vi "convert type defs to channels.vi"() -> (0 "error out":errorcluster, 3 "Array out":refnum<class "TBM channel.lvclass">[](array[class]))   [LabVIEW 2013, in "fixed channel tag bus module configuration.lvclass"]
uses:
  fixed channel tag bus module configuration.lvclass
  <vilib>/NI/Tag Bus Module Framework/channel/TBM channel.lvclass
  <vilib>/NI/Tag Bus Module Framework/channel/channel classification.ctl
  <vilib>/regexp/Match Regular Expression.xnode
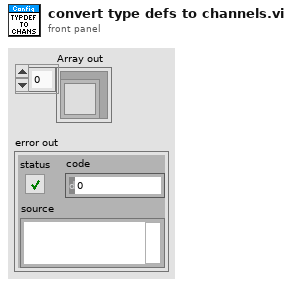
[diagram p1: front panel]
types:
  T1 = typedef "TBM channel.lvclass/channel classification.ctl" = enum16{"input data", "output data", "processing parameter", "processing result"}
  T2 = typedef "tag bus.lvlib/tag descriptor.lvclass/Data Type.ctl" = enum16{"Double", "Single", "I64", "I32", "I16", "I8", "U64", "U32", "U16", "U8", "Boolean", "String", "Array of Double", "Array of Single", "Array of I64", "Array of I32", "Array of I16", "Array of I8", "Array of U64", "Array of U32", "Array of U16", "Array of U8", "Array of Boolean", "Array of String"}
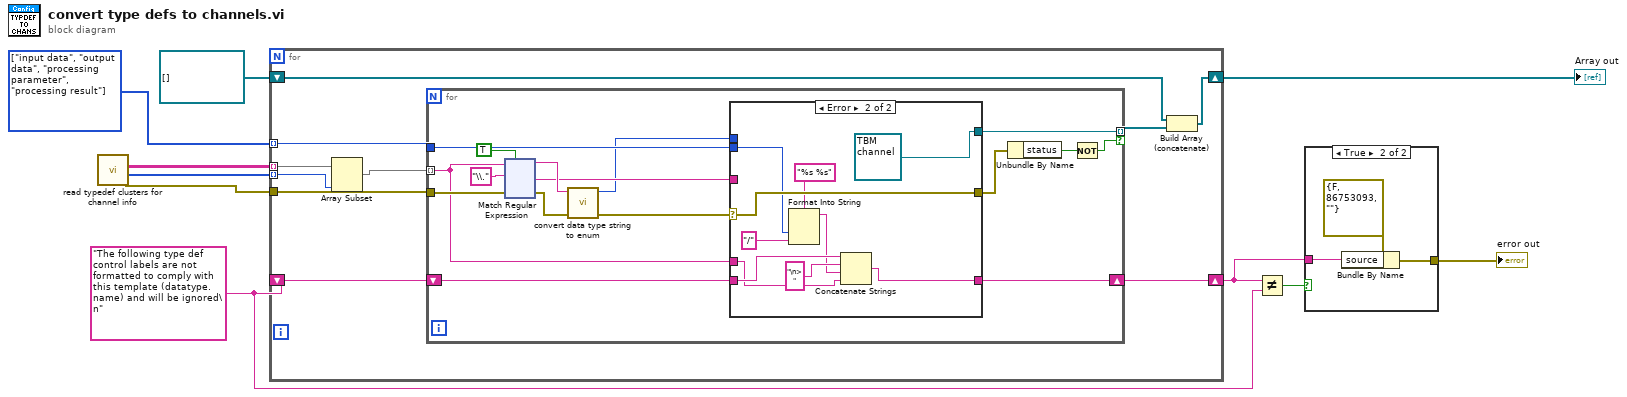
[diagram p0: block diagram]
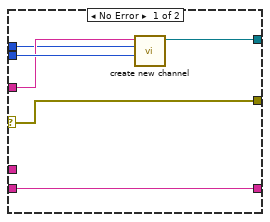
[diagram p3: hidden frame]
diagram:
  w2 = T1[] [enum."input data", enum."output data", enum."processing parameter", enum."processing result"] items=["input data", "output data", "processing parameter", "processing result"]
  w7 = "The following type def control labels are not formatted to comply with this template (datatype.name) and will be ignored\n"
  n1 = call "read typedef clusters for channel info.vi"() -> ("error out"=w5:errorcluster, "Channel Counts"=w1:i32[], "> Categorized name list >"=w4:string[][])  [unwired: 8 in, 1 out]
  n2 = for {
    tunnel: w2 -> [w20] mode=indexing
    shift-right: [w18] -> w6
    shift-left: refnum<class "TBM channel.lvclass">[] [] -> [w17]
    tunnel: w4 -> [w13] mode=indexing
    tunnel: w5 -> [w16]
    shift-right: [w14] -> w9
    shift-left: w7 -> [w15]
    tunnel: w1 -> [w12] mode=indexing
    n3 = Array Subset(array=w13, length=w12) -> (w11:string[])  [unwired: 1 in]
    n4 = for {
      tunnel: w20 -> [w35]
      tunnel: [w36] -> w19 mode=indexing if=w26
      tunnel: w11 -> [w23] mode=indexing
      shift-right: [w21] -> w14
      shift-left: w15 -> [w22]
      tunnel: w16 -> [w32]
      n5 = xnode "Match Regular Expression"("input string"=w23, "regular expression"="\\.", "error in"=w32, "ignore case? (F)"=TRUE) -> ("before match"=w30:string, "after match"=w29:string, "error out"=w31:errorcluster)  [unwired: 2 in, 2 out]
      n6 = call "convert data type string to enum.vi"("error in"=w31, "Data Type String"=w30) -> ("error out"=w28:errorcluster, "Data Type Enum"=w24:T2)  [unwired: 8 in]
      n7 = case shown="Error" w28 {
        selector: w28 -> [w154 w165]
        tunnel: w35 -> [w156 w161]
        tunnel: [w154 w165] -> w27
        tunnel: [w155 refnum<class "TBM channel.lvclass"> refnum ("channel")] -> w36
        tunnel: w29 -> [w153 _]
        tunnel: w24 -> [w152 _]
        tunnel: w23 -> [_ w157]
        tunnel: w22 -> [w151 w164]
        tunnel: [w151 w163] -> w21
        frame No Error {
          n8 = call <vilib>:"create new channel.vi"("channel classification"=w156, "data type"=w152, "channel name"=w153) -> ("channel"=w155:refnum<class "TBM channel.lvclass">)  [unwired: 8 in]
        }
        frame Error {
          n9 = Format Into String(format string="%s %s", w161, "/") -> (resulting string=w158:string)  [unwired: 2 in, 1 out]
          n10 = Concatenate Strings(w164, "\n> " ("string"), w158, w157) -> (w163:string)
        }
      }
      n11 = Unbundle By Name(w27) -> ("status"=w25:bool)
      n12 = Not(x=w25) -> (.not. x?=w26:bool)
    }
    n13 = Build Array (concatenate)(w17, w19) -> (w18:refnum<class "TBM channel.lvclass">[])
  }
  "Array out" <- w6
  n14 = Not Equal?(x=w9, y=w7) -> (x != y?=w8:bool)
  n15 = case shown="True" w8 {
    tunnel: w9 -> [_ w168]
    tunnel: [_ w167] -> w10
    frame False {
    }
    frame True {
      n16 = Bundle By Name(cluster=errorcluster {"status"=FALSE, "code"=86753093, "source"=""} ("error constant"), "source"=w168) -> (w167:errorcluster)
    }
  }
  "error out" <- w10
